vi "RIMAS Detector FITS hdr update detector settings.vi"(8 "Error In":errorcluster, 10 "FITS Detector Settings":T1, 11 "fits hdr":string[](array[string])) -> (0 "Error Out":errorcluster, 3 "fits hdr out":string[](array[string]))   [LabVIEW 2022 SP3]
uses:
  RIMAS Observation Config.ctl
  FITS/FITS hdr update field dbl.vi
panel:
  # "sec"
  # "sec"
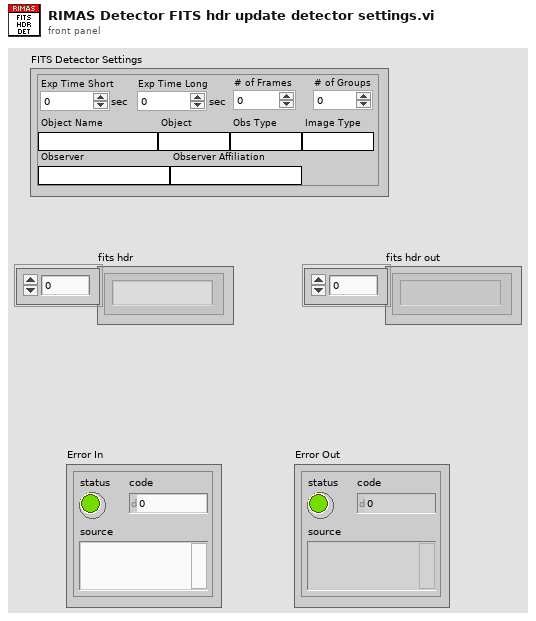
[diagram p1: front panel]
types:
  T1 = typedef "RIMAS Observation Config.ctl" = cluster{"Exp Time Short":dbl, "# of Frames":dbl, "Exp Time Long":dbl, "# of Groups":dbl, "Object Name":string, "Object":string, "Obs Type":string, "Image Type":string, "Observer":string, "Observer Affiliation":string}
  T2 = cluster{"Date/time":string, "run number":u16, "last steps made":i32, "total steps":i32, "position steps":i32, "Slot filter number":i32, "filter /stage name":string}
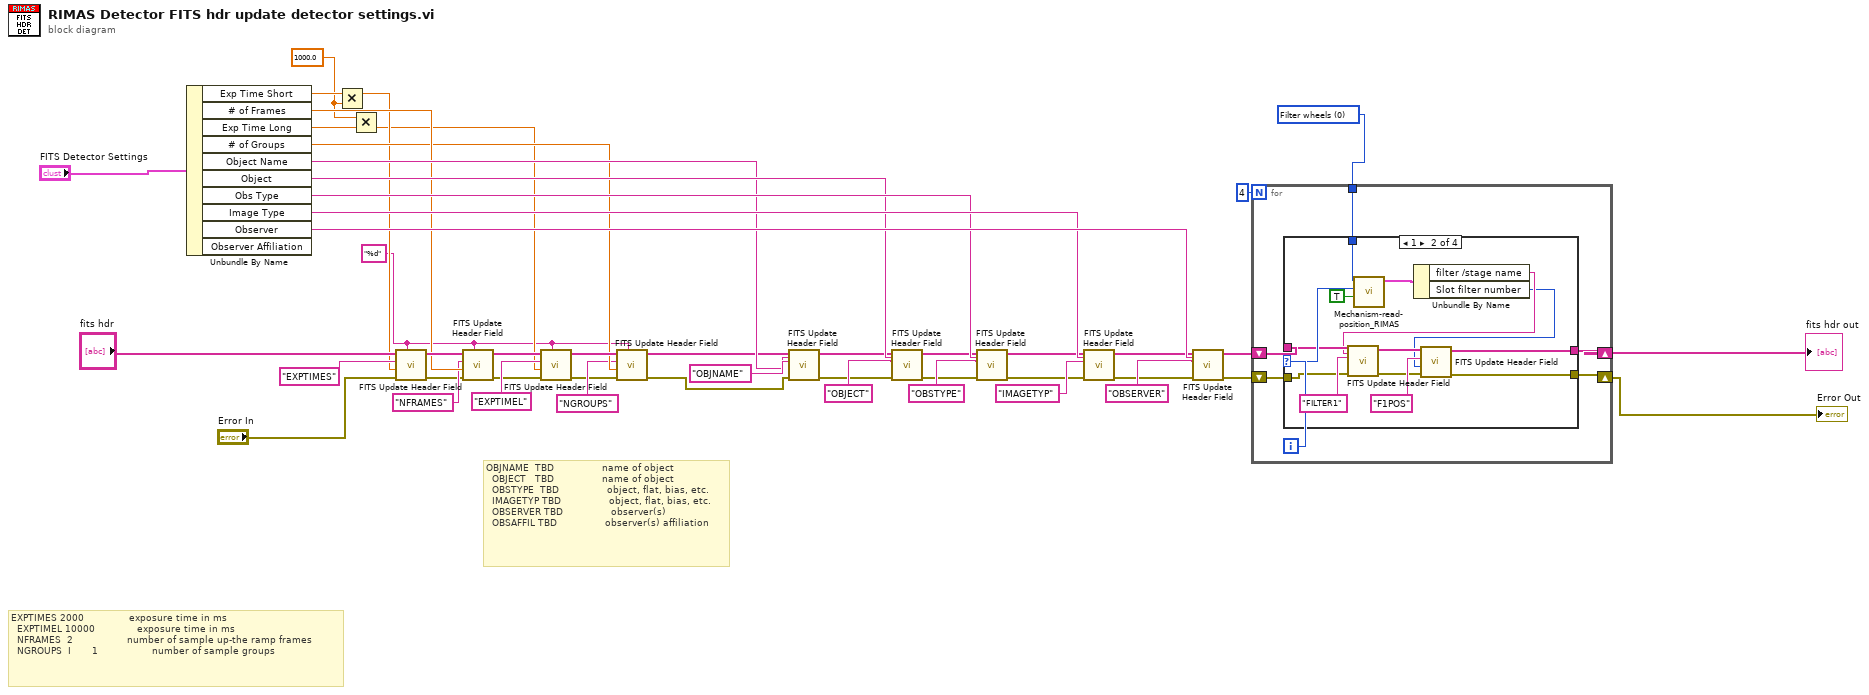
[diagram p0: block diagram]
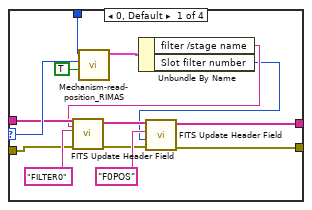
[diagram p2: hidden frame]
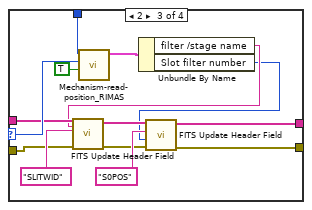
[diagram p3: hidden frame]
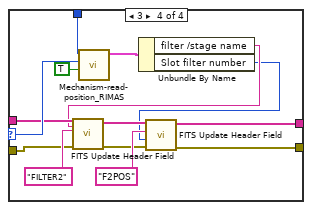
[diagram p4: hidden frame]
diagram:
  w1 = u16 0 items=["Filter wheels", "Focus"] ("Mechanism type")
  w7 = "%d" ("Format")
  w8 = 1000.0 ("y")
  # "EXPTIMES 2000               exposure time in ms\n  EXPTIMEL 10000              exposure time in ms\n  NFRAMES  2                  number of sample up-the ramp frames\n  NGROUPS  I       1                  number of sample groups"
  # "OBJNAME  TBD                name of object\n  OBJECT   TBD                name of object\n  OBSTYPE  TBD                object, flat, bias, etc.\n  IMAGETYP TBD                object, flat, bias, etc.\n  OBSERVER TBD                observer(s) \n  OBSAFFIL TBD                observer(s) affiliation"
  n1 = Unbundle By Name("FITS Detector Settings") -> ("Exp Time Short"=w30:dbl, "# of Frames"=w25:dbl, "Exp Time Long"=w24:dbl, "# of Groups"=w23:dbl, "Object Name"=w37:string, "Object"=w39:string, "Obs Type"=w41:string, "Image Type"=w43:string, "Observer"=w45:string)  [unwired: 1 out]
  n2 = Multiply(x=w30, y=w8) -> (x*y=w10:dbl)
  n3 = Multiply(x=w8, y=w24) -> (x*y=w9:dbl)
  n4 = call-poly "FITS Update Header Field.vi"("Format"=w7, "Error In"="Error In", "Value"=w10, "Field"="EXPTIMES", "fits hdr"="fits hdr") -> ("Error Out"=w18:errorcluster, "fits hdr out"=w29:string[])  [unwired: 5 in]
  n5 = call-poly "FITS Update Header Field.vi"("Format"=w7, "Error In"=w18, "Value"=w25, "Field"="NFRAMES", "fits hdr"=w29) -> ("Error Out"=w17:errorcluster, "fits hdr out"=w28:string[])  [unwired: 5 in]
  n6 = call-poly "FITS Update Header Field.vi"("Format"=w7, "Error In"=w17, "Value"=w9, "Field"="EXPTIMEL", "fits hdr"=w28) -> ("Error Out"=w16:errorcluster, "fits hdr out"=w27:string[])  [unwired: 5 in]
  n7 = call-poly "FITS Update Header Field.vi"("Format"=w7, "Error In"=w16, "Value"=w23, "Field"="NGROUPS", "fits hdr"=w27) -> ("Error Out"=w15:errorcluster, "fits hdr out"=w26:string[])  [unwired: 5 in]
  n8 = call-poly "FITS Update Header Field.vi"("Format"=w37, "Error In"=w15, "Field"="OBJNAME", "fits hdr"=w26) -> ("Error Out"=w14:errorcluster, "fits hdr out"=w36:string[])  [unwired: 6 in]
  n9 = call-poly "FITS Update Header Field.vi"("Format"=w39, "Error In"=w14, "Field"="OBJECT", "fits hdr"=w36) -> ("Error Out"=w13:errorcluster, "fits hdr out"=w35:string[])  [unwired: 6 in]
  n10 = call-poly "FITS Update Header Field.vi"("Format"=w41, "Error In"=w13, "Field"="OBSTYPE", "fits hdr"=w35) -> ("Error Out"=w12:errorcluster, "fits hdr out"=w34:string[])  [unwired: 6 in]
  n11 = call-poly "FITS Update Header Field.vi"("Format"=w43, "Error In"=w12, "Field"="IMAGETYP", "fits hdr"=w34) -> ("Error Out"=w11:errorcluster, "fits hdr out"=w33:string[])  [unwired: 6 in]
  n12 = call-poly "FITS Update Header Field.vi"("Format"=w45, "Error In"=w11, "Field"="OBSERVER", "fits hdr"=w33) -> ("Error Out"=w5:errorcluster, "fits hdr out"=w6:string[])  [unwired: 6 in]
  n13 = for {
    N: 4 -> [_]
    shift-right: [w49] -> w3
    shift-left: w5 -> [w51]
    shift-right: [w48] -> w2
    shift-left: w6 -> [w52]
    tunnel: w1 -> [w50]
    i -> [w53]
    n14 = case shown="1" w53 {
      selector: w53 -> [w66 w80 w94 w108]
      tunnel: w52 -> [w61 w75 w89 w103]
      tunnel: w51 -> [w59 w73 w87 w101]
      tunnel: w50 -> [w67 w81 w95 w109]
      tunnel: [w57 w71 w85 w99] -> w49
      tunnel: [w56 w70 w84 w98] -> w48
      frame 0, Default {
        n15 = call "Mechanism-read-position_RIMAS.vi"("Enable empty file warning"=TRUE, "Mechanism  number"=w66, "Mechanism type"=w67) -> ("Position data"=w64:T2)  [unwired: 3 in, 5 out]
        n16 = Unbundle By Name(w64) -> ("filter /stage name"=w55:string, "Slot filter number"=w54:i32)
        n17 = call-poly "FITS Update Header Field.vi"("Format"=w55, "Error In"=w59, "Field"="FILTER0", "fits hdr"=w61) -> ("Error Out"=w58:errorcluster, "fits hdr out"=w60:string[])  [unwired: 6 in]
        n18 = call-poly "FITS Update Header Field.vi"("Error In"=w58, "Value"=w54, "Field"="F0POS", "fits hdr"=w60) -> ("Error Out"=w57:errorcluster, "fits hdr out"=w56:string[])  [unwired: 6 in]
      }
      frame 1 {
        n19 = call "Mechanism-read-position_RIMAS.vi"("Enable empty file warning"=TRUE, "Mechanism  number"=w80, "Mechanism type"=w81) -> ("Position data"=w78:T2)  [unwired: 3 in, 5 out]
        n20 = Unbundle By Name(w78) -> ("filter /stage name"=w69:string, "Slot filter number"=w68:i32)
        n21 = call-poly "FITS Update Header Field.vi"("Format"=w69, "Error In"=w73, "Field"="FILTER1", "fits hdr"=w75) -> ("Error Out"=w72:errorcluster, "fits hdr out"=w74:string[])  [unwired: 6 in]
        n22 = call-poly "FITS Update Header Field.vi"("Error In"=w72, "Value"=w68, "Field"="F1POS", "fits hdr"=w74) -> ("Error Out"=w71:errorcluster, "fits hdr out"=w70:string[])  [unwired: 6 in]
      }
      frame 2 {
        n23 = call "Mechanism-read-position_RIMAS.vi"("Enable empty file warning"=TRUE, "Mechanism  number"=w94, "Mechanism type"=w95) -> ("Position data"=w92:T2)  [unwired: 3 in, 5 out]
        n24 = Unbundle By Name(w92) -> ("filter /stage name"=w83:string, "Slot filter number"=w82:i32)
        n25 = call-poly "FITS Update Header Field.vi"("Format"=w83, "Error In"=w87, "Field"="SLITWID", "fits hdr"=w89) -> ("Error Out"=w86:errorcluster, "fits hdr out"=w88:string[])  [unwired: 6 in]
        n26 = call-poly "FITS Update Header Field.vi"("Error In"=w86, "Value"=w82, "Field"="S0POS", "fits hdr"=w88) -> ("Error Out"=w85:errorcluster, "fits hdr out"=w84:string[])  [unwired: 6 in]
      }
      frame 3 {
        n27 = call "Mechanism-read-position_RIMAS.vi"("Enable empty file warning"=TRUE, "Mechanism  number"=w108, "Mechanism type"=w109) -> ("Position data"=w106:T2)  [unwired: 3 in, 5 out]
        n28 = Unbundle By Name(w106) -> ("filter /stage name"=w97:string, "Slot filter number"=w96:i32)
        n29 = call-poly "FITS Update Header Field.vi"("Format"=w97, "Error In"=w101, "Field"="FILTER2", "fits hdr"=w103) -> ("Error Out"=w100:errorcluster, "fits hdr out"=w102:string[])  [unwired: 6 in]
        n30 = call-poly "FITS Update Header Field.vi"("Error In"=w100, "Value"=w96, "Field"="F2POS", "fits hdr"=w102) -> ("Error Out"=w99:errorcluster, "fits hdr out"=w98:string[])  [unwired: 6 in]
      }
    }
  }
  "Error Out" <- w3
  "fits hdr out" <- w2
